vi "rad_Refresh Target Information.vi"(7 "Reduce Discovery Timeout":bool=TRUE, 8 "error in (no error)":errorcluster, 10 "User Added Targets Only":bool, 11 "User Added Targets":string[](array[string])) -> (0 "error out":errorcluster, 3 "Targets Information":T1[](array[typedef]) {"Primary NIC"."IP Address Request Mode" items=["Static"=1, "DHCP/Link-Local"=2, "Link-Local Only"=4, "DHCP Only"=8]})   [LabVIEW 2016]
uses:
  TypeDefs/rad_Target Information.ctl
  TypeDefs/rad_Target Network Settings.ctl
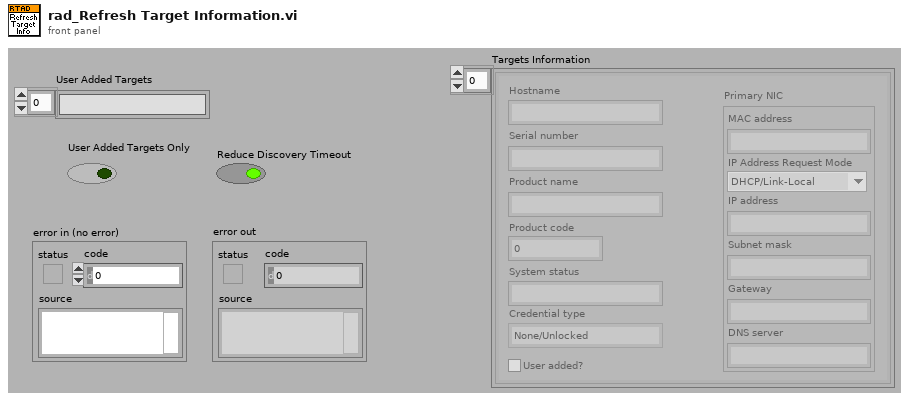
[diagram p1: front panel]
types:
  T1 = typedef "rad_Target Information.ctl" = cluster{"Hostname":string, "Serial number":string, "Product name":string, "Product code":i32, "System status":string, "Credential type":enum16{"None/Unlocked", "FTP Password", "NIAuth Credentials"}, "User added?":bool, "Primary NIC":T2}
  T2 = typedef "rad_Target Network Settings.ctl" = cluster{"MAC address":string, "IP Address Request Mode":i32, "IP address":string, "Subnet mask":string, "Gateway":string, "DNS server":string}
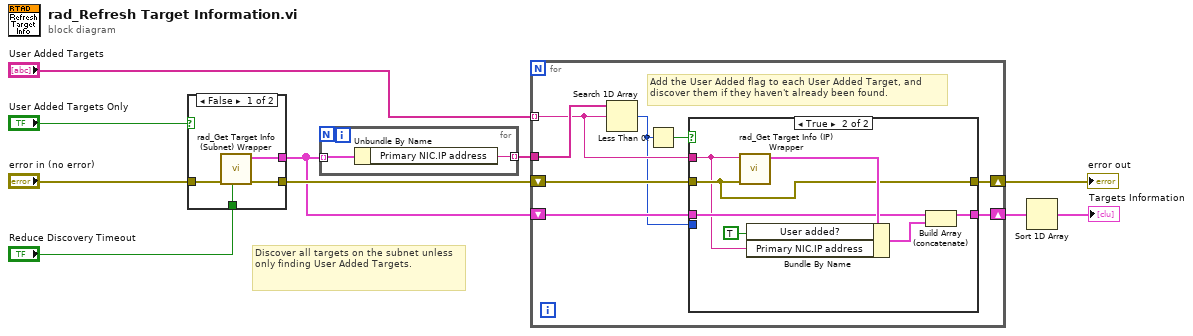
[diagram p0: block diagram]
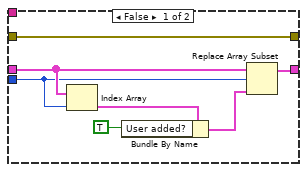
[diagram p2: hidden frame]
diagram:
  # "Discover all targets on the subnet unless only finding User Added Targets."
  n1 = case shown="False" "User Added Targets Only" {
    tunnel: "error in (no error)" -> [w14 w15]
    tunnel: [w13 _] -> w5
    tunnel: [w12 w15] -> w8
    tunnel: "Reduce Discovery Timeout" -> [w11 _]
    frame False {
      n2 = call "rad_Get Target Info (Subnet) Wrapper.vi"("reduce discovery timeout (T)"=w11, "error in (no error)"=w14) -> ("error out"=w12:errorcluster, "target information"=w13:T1[])  [unwired: 8 in]
    }
    frame True {
    }
  }
  n3 = for {
    tunnel: w5 -> [w17] mode=indexing
    tunnel: [w16] -> w6 mode=indexing
    n4 = Unbundle By Name(w17) -> ("Primary NIC.IP address"=w16:string)
  }
  n5 = for {
    tunnel: "User Added Targets" -> [w22] mode=indexing
    tunnel: w6 -> [w24]
    shift-right: [w19] -> w4
    shift-left: w5 -> [w21]
    shift-right: [w18] -> w3
    shift-left: w8 -> [w25]
    # "Add the User Added flag to each User Added Target, and discover them if they haven't already been found."
    n6 = Search 1D Array(1D array=w24, element=w22) -> (index of element=w20:i32)  [unwired: 1 in]
    n7 = Less Than 0?(x=w20) -> (x < 0?=w23:bool)
    n8 = case shown="True" w23 {
      tunnel: w25 -> [w32 w34]
      tunnel: w22 -> [_ w33]
      tunnel: [w32 w34] -> w18
      tunnel: w21 -> [w29 w36]
      tunnel: w20 -> [w26 _]
      tunnel: [w28 w35] -> w19
      frame False {
        n9 = Index Array(array=w29, index=w26) -> (element=w31:T1)
        n10 = Bundle By Name(cluster=w31, "User added?"=TRUE ("User Added?")) -> (w27:T1)
        n11 = Replace Array Subset(array=w29, new element=w27, index=w26) -> (w28:T1[])
      }
      frame True {
        n12 = call "rad_Get Target Info (IP) Wrapper.vi"("error in (no error)"=w34, "target address"=w33) -> ("Target settings"=w39:T1)  [unwired: 8 in, 1 out]
        n13 = Bundle By Name(cluster=w39, "User added?"=TRUE ("User Added?"), "Primary NIC.IP address"=w33) -> (w37:T1)
        n14 = Build Array (concatenate)(w36, w37) -> (w35:T1[])
      }
    }
  }
  "error out" <- w3
  n15 = Sort 1D Array(array=w4) -> (sorted array=→"Targets Information":T1[])
